vi "Sensor_Reads.vi"() -> ()   [LabVIEW 2020]
uses:
  <vilib>/Rock Robotics/WPI/ThirdParty/Phoenix-LabVIEW/Pigeon IMU/CTRE_PigeonIMU_TareType.ctl
  <vilib>/Rock Robotics/Network Tables/NT Read Number.vi
  Globals/Sensor_Values.vi
  Hardware/Drive/Drive_Hardware_Globals.vi
  Globals/Drive_Globals.vi
  <vilib>/Rock Robotics/Network Tables/NT Write Number.vi
  <vilib>/Rock Robotics/WPI/ThirdParty/Phoenix-LabVIEW/Pigeon IMU/CTRE_PigeonIMU_GetYPR.vi
  <vilib>/Rock Robotics/WPI/ThirdParty/Phoenix-LabVIEW/Motor Controller/Get/CTRE_Phoenix_MotorController_GetSelectedSensorData.vi
  Hardware/Climber/Climber_Hardware_Globals.vi
  <vilib>/Rock Robotics/WPI/ThirdParty/Phoenix-LabVIEW/CANCoder/Set/CTRE_Phoenix_CANcoder_SetPosition.vi
  Globals/Calibration_And_Constant_Globals.vi
  <vilib>/Rock Robotics/WPI/ThirdParty/Phoenix-LabVIEW/CANCoder/Get/CTRE_Phoenix_CANcoder_GetSensorData.vi
  Hardware/Cowl/Cowl_Hardware_Globals.vi
  Globals/Magazine_Globals.vi
  <vilib>/Rock Robotics/WPI/Utilities/WPI_GetSetVariantRefNum.vi
  Hardware/Flywheel/Flywheel_Hardware_Globals.vi
  Hardware/Turret/Turret_Hardware_Globals.vi
  <vilib>/Rock Robotics/WPI/ThirdParty/Phoenix-LabVIEW/Motor Controller/Get/CTRE_Phoenix_MotorController_GetPulseWidthAll.vi
  <vilib>/Rock Robotics/Network Tables/NT Read Boolean.vi
  Globals/Funnel_global.vi
  <vilib>/Rock Robotics/WPI/ThirdParty/Phoenix-LabVIEW/CANCoder/Set/CTRE_Phoenix_CANcoder_SetPositionToAbsolute.vi
  <vilib>/Rock Robotics/WPI/ThirdParty/Phoenix-LabVIEW/Motor Controller/Get/CTRE_Phoenix_MotorController_GetSupplyAndStatorCurrent_Enhanced.vi
panel:
  out "safe_to_move_turret?":bool
  in  "safe inner arm position for turret":i32
  in  "disable_limit_switch_zero_thing":bool
  out "Outer_Arm_Limit_Switch":bool=TRUE
  out "outer arm pulse width":i32
  out "inner arm pulse width":i32=578
  in  "inner arm pivot zero (ticks)":i32=-1151
  in  "outer arm pivot zero (ticks)":i32=921
  in  "reset_turret_position":bool
  out "turret position":i32
  in  "reset_cowl_position":bool
  in  "Cowl_Zero(deg)":dbl=61.6
  out "ball in funnel":bool
  in  "funnel current detect threshold":dbl=35.0
  in  "mag IR threshold":dbl=1.7
  out "limelight_distance_to_target":dbl=240.7612770897626
  out "Funnel_Supply_Current":dbl(graph)
  out "Mag IR Voltage":dbl=0.306396453
  in  "limelight mounting angle (deg)":dbl=36.64
  in  "height of the target (in)":dbl=104.0
  in  "height of robot (in)":dbl=37.625
  in  "Front_Right_Zero":dbl[](array[numeric])=[99.4, 331.43]
  out "front right raw":dbl=146.865234375
  out "FR mod":dbl=146.865234375
  in  "Front_Left_Zero":dbl[](array[numeric])=[338.818, 288.54]
  out "front left raw":dbl=111.357421875
  out "FL mod":dbl=111.357421875
  in  "Back_Left_Zero":dbl[](array[numeric])=[255.059, 271.84]
  out "back left raw":dbl=93.427734375
  out "BL mod":dbl=93.427734375
  in  "Back_Right_Zero":dbl[](array[numeric])=[182.197, 189.4]
  out "back right raw":dbl=195.29296875
  out "BR mod":dbl=195.29296875
  # "0th index is alpha, 1st index is beta"
  # "e"
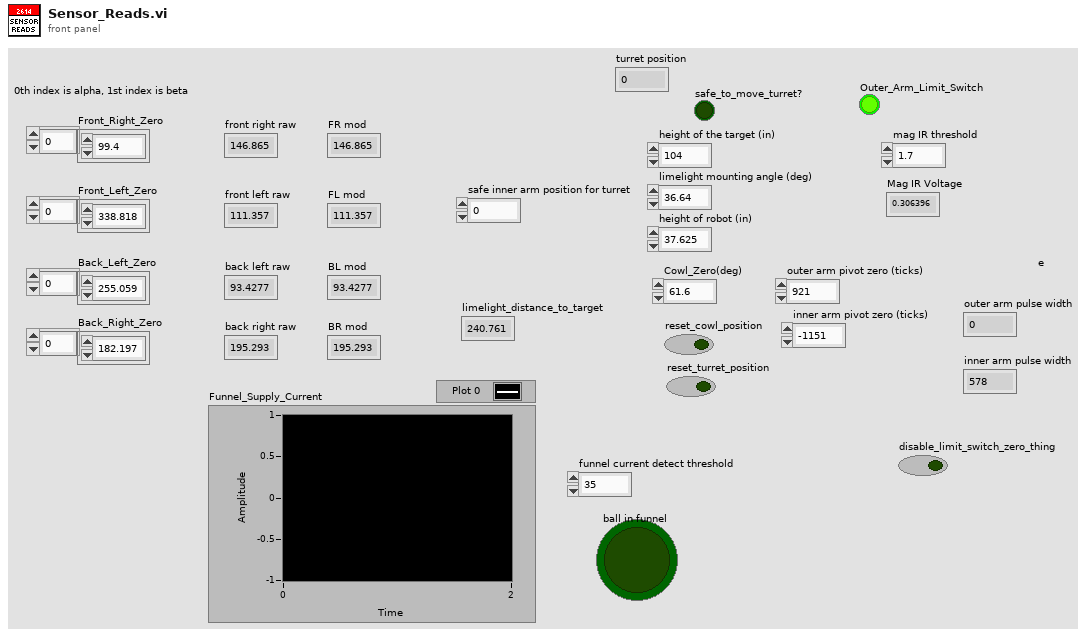
[diagram p1: front panel]
types:
  T1 = typedef "WPI_MotorControlDeviceRef.ctl" = cluster{"DeviceStatus":errorcluster, "Type":T2, "PWM":cluster{"PWM Channel":T3, "DeadBand":T4}, "CAN":cluster{"Device Number":u8, "SetOutput VI Ref":variant, "GetOutput VI Ref":variant, "Enable VI Ref":variant, "Disable VI Ref":variant, "Data":variant}, "Invert":bool, "DIO PWM":cluster{"PWM \"Enable\" Channel":T3, "DIOChannel":T5, "PWM Rate":dbl}}
  T2 = typedef "WPI_MotorControlType.ctl" = enum16{"PWM", "CAN", "DIO PWM"}
  T3 = typedef "FPGA_DIOPWMChannel.ctl" = enum8{"PWM 0", "PWM 1", "PWM 2", "PWM 3", "PWM 4", "PWM 5", "PWM 6", "PWM 7", "PWM 8", "PWM 9", "PWM MXP 0", "PWM MXP 1", "PWM MXP 2", "PWM MXP 3", "PWM MXP 4", "PWM MXP 5", "PWM MXP 6", "PWM MXP 7", "PWM MXP 8", "PWM MXP 9", "Invalid"}
  T4 = typedef "WPI_PWMDeadband.ctl" = cluster{"Name":string, "maxPositivePwm":i32, "minPositivePwm":i32, "centerPwm":i32, "maxNegativePwm":i32, "minNegativePwm":i32, "angularRange":u16}
  T5 = typedef "FPGA_DIOChannel.ctl" = enum8{"DIO 0", "DIO 1", "DIO 2", "DIO 3", "DIO 4", "DIO 5", "DIO 6", "DIO 7", "DIO 8", "DIO 9", "DIO MXP 0", "DIO MXP 1", "DIO MXP 2", "DIO MXP 3", "DIO MXP 4", "DIO MXP 5", "DIO MXP 6", "DIO MXP 7", "DIO MXP 8", "DIO MXP 9", "DIO MXP 10", "DIO MXP 11", "DIO MXP 12", "DIO MXP 13", "DIO MXP 14", "DIO MXP 15", "SPI Port CS1", "SPI Port CS2", "SPI Port CS3", "SPI Port MISO", "SPI Port MOSI", "Invalid"}
  T6 = typedef "CTRE_Phoenix_CANcoder_DeviceRef.ctl" = cluster{"DeviceStatus":errorcluster, "Device Number":u8, "Handle":u64, "UsageFrame":u32, "Library Path":path}
  T7 = typedef "CTRE_PigeonIMU_DeviceRef.ctl" = cluster{"DeviceStatus":errorcluster, "Device Number":u8, "Type":T8, "Device ID":u32, "Handle":u64, "UsageFrame":u32, "Library Path":path}
  T8 = typedef "CTRE_PigeonIMU_ConnectionType.ctl" = u32
  T9 = typedef "WPI_DigitalInputDevRef.ctl" = cluster{"DevStatus":errorcluster, "DIO Channel":T5}
  T10 = typedef "WPI_AnalogChannelDevRef.ctl" = cluster{"DevStatus":errorcluster, "Analog Channel":T11}
  T11 = typedef "FPGA_AIChannel.ctl" = enum8{"AI 0", "AI 1", "AI 2", "AI 3", "AI MXP 0", "AI MXP 1", "AI MXP 2", "AI MXP 3", "Invalid"}
  T12 = typedef "CTRE_PigeonIMU_TareType.ctl" = u8
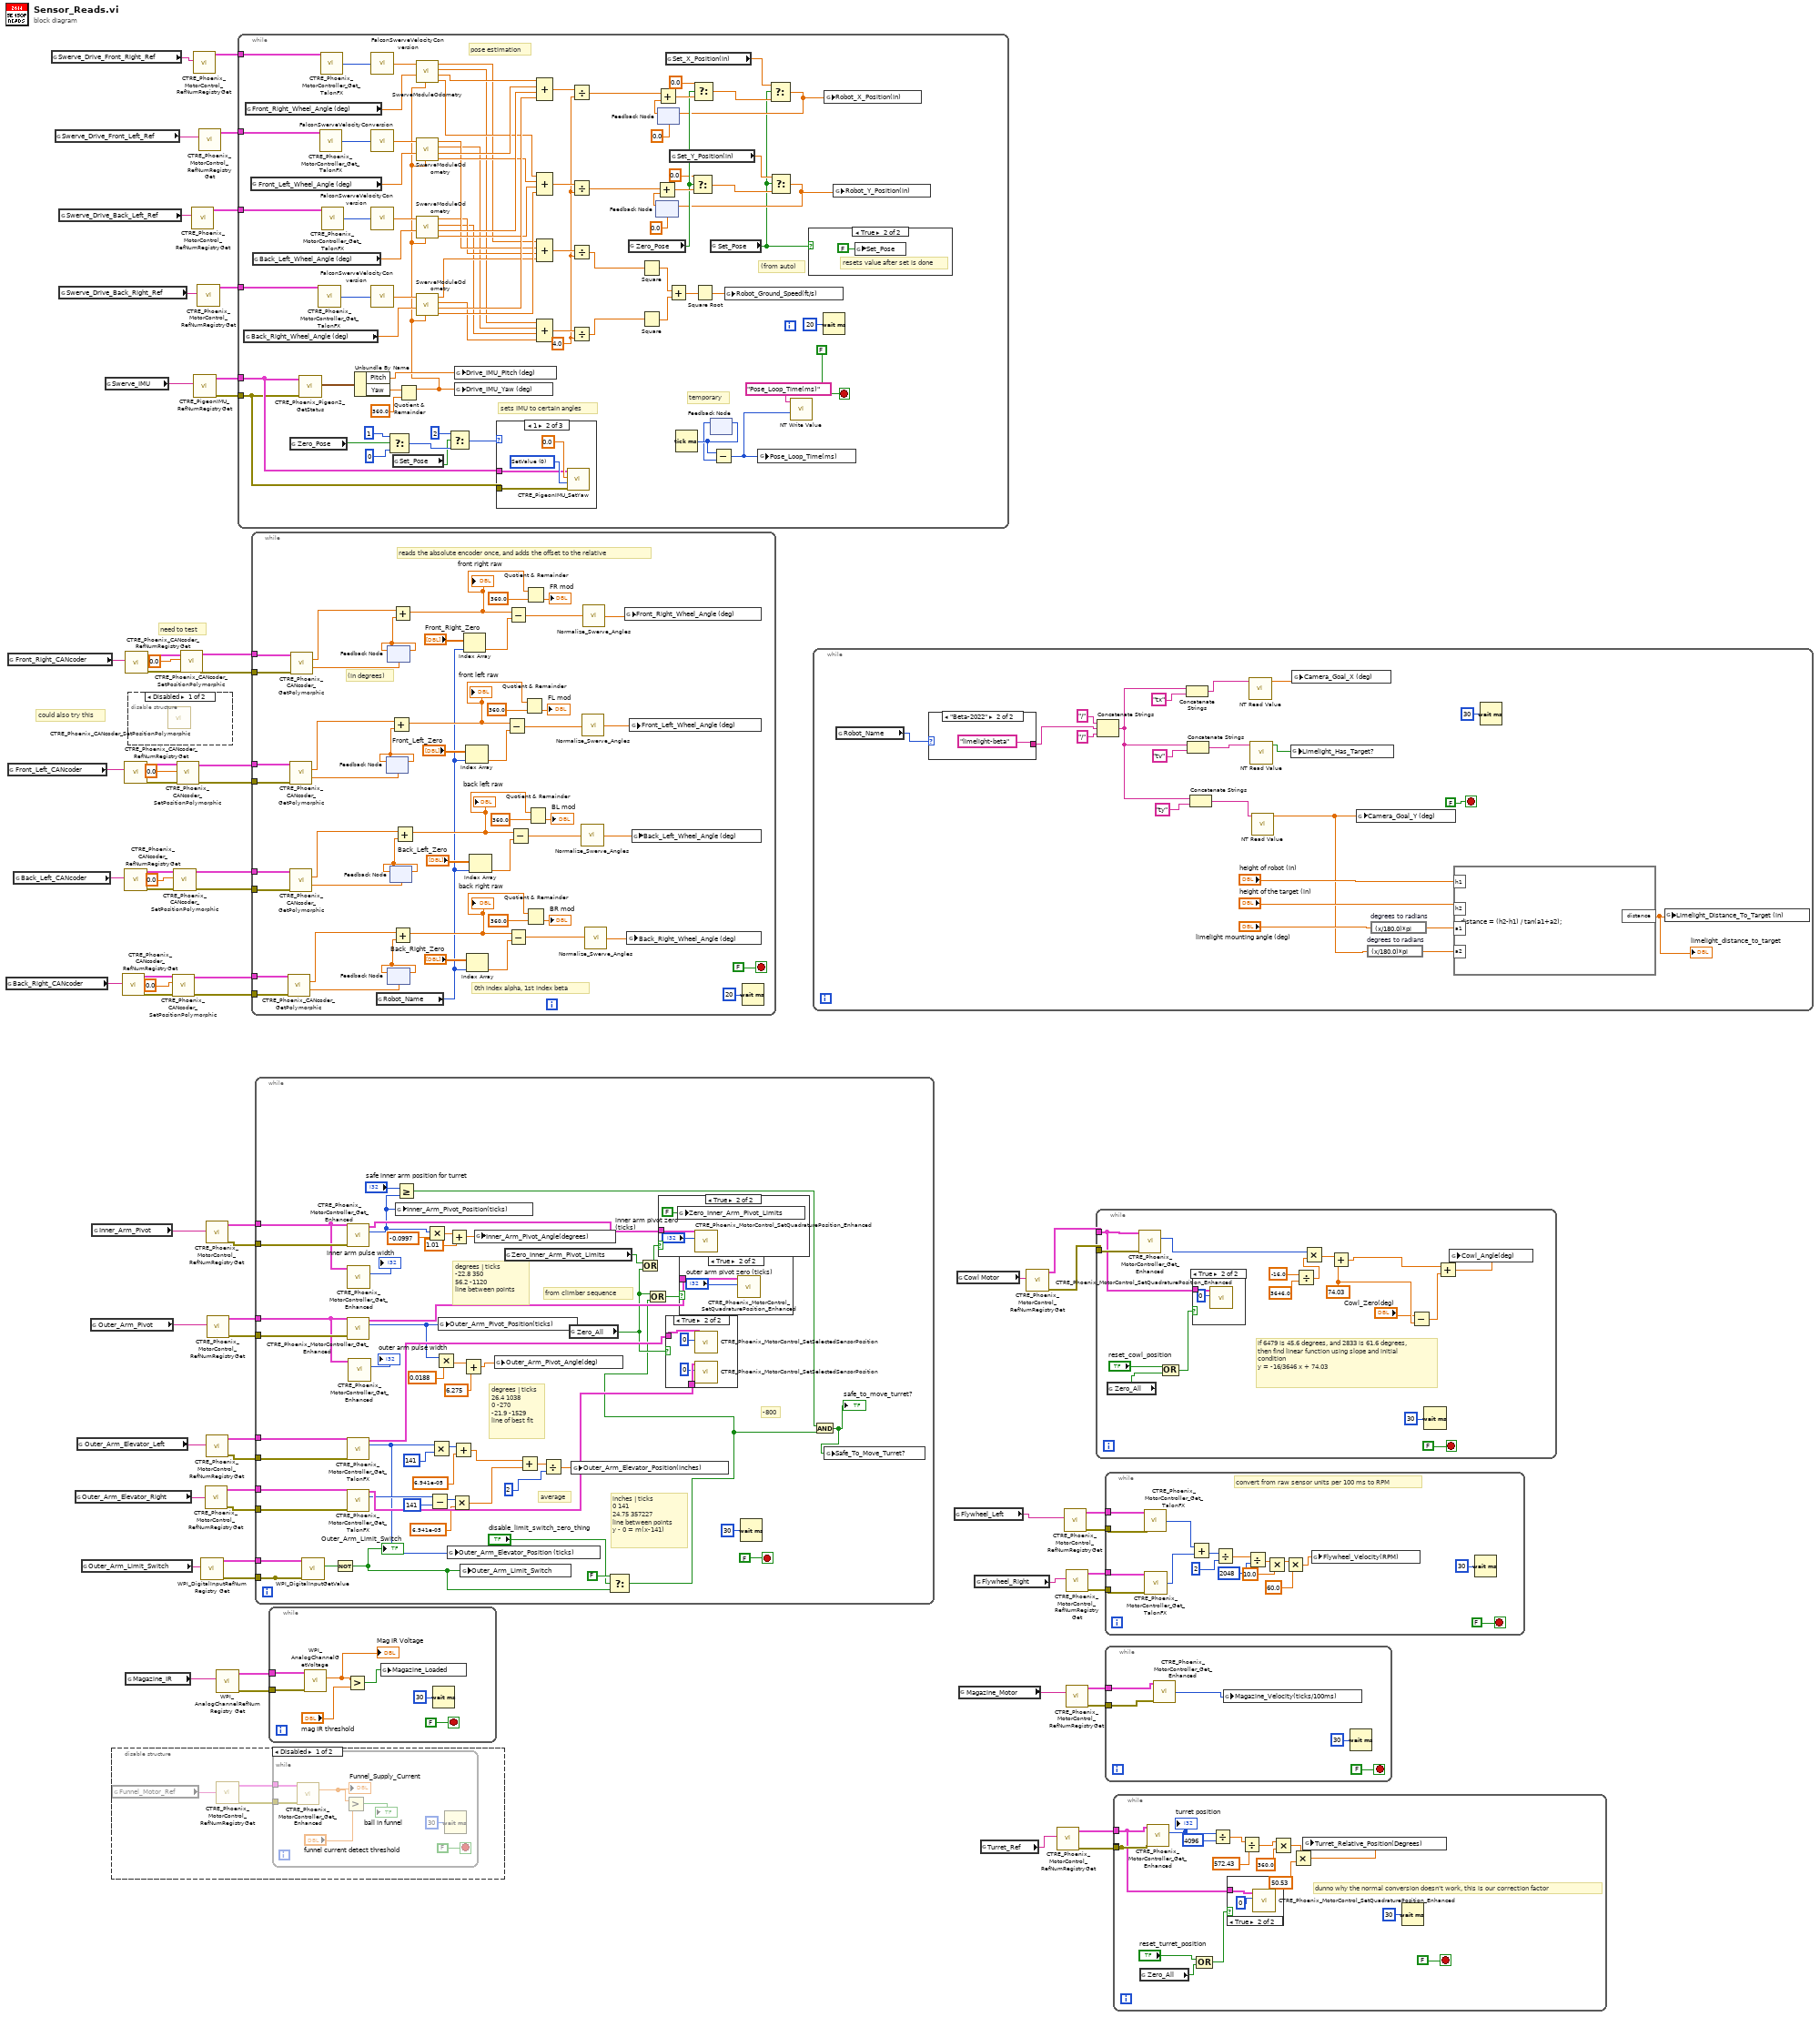
[diagram p0: block diagram]
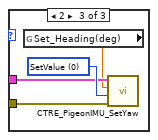
[diagram p10: hidden frame]
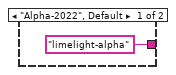
[diagram p12: hidden frame]
diagram:
  # "could also try this"
  # "need to test"
  n1 = global read "Drive_Hardware_Globals.vi" "Back_Right_CANcoder"() -> (w54:string)
  n2 = global read "Drive_Hardware_Globals.vi" "Front_Right_CANcoder"() -> (w57:string)
  n3 = global read "Drive_Hardware_Globals.vi" "Front_Left_CANcoder"() -> (w56:string)
  n4 = global read "Drive_Hardware_Globals.vi" "Back_Left_CANcoder"() -> (w55:string)
  n5 = global read "Drive_Hardware_Globals.vi" "Swerve_Drive_Front_Right_Ref"() -> (w58:string)
  n6 = global read "Drive_Hardware_Globals.vi" "Swerve_Drive_Front_Left_Ref"() -> (w59:string)
  n7 = global read "Drive_Hardware_Globals.vi" "Swerve_Drive_Back_Left_Ref"() -> (w68:string)
  n8 = global read "Drive_Hardware_Globals.vi" "Swerve_Drive_Back_Right_Ref"() -> (w67:string)
  n9 = global read "Climber_Hardware_Globals.vi" "Outer_Arm_Elevator_Right"() -> (w32:string)
  n10 = global read "Climber_Hardware_Globals.vi" "Outer_Arm_Elevator_Left"() -> (w33:string)
  n11 = global read "Climber_Hardware_Globals.vi" "Outer_Arm_Limit_Switch"() -> (w3:string)
  n12 = global read "Climber_Hardware_Globals.vi" "Outer_Arm_Pivot"() -> (w22:string)
  n13 = global read "Climber_Hardware_Globals.vi" "Inner_Arm_Pivot"() -> (w31:string)
  n14 = global read "Drive_Hardware_Globals.vi" "Swerve_IMU"() -> (w62:string)
  n15 = disable-structure shown="Disabled" {
    frame Disabled {
      n16 = global read "Funnel_global.vi" "Funnel_Motor_Ref"() -> (w71:string)
      n17 = call <vilib>:"CTRE_Phoenix_MotorControl_RefNumRegistryGet.vi"("refnum name"=w71) -> ("error out"=w69:errorcluster, "PhoenixMotorControlDevRef"=w70:T1)  [unwired: 9 in]
      n18 = while {
        tunnel: w70 -> [w76]
        tunnel: w69 -> [w75]
        stop <- FALSE stop-if-true
        n19 = call-poly <vilib>:"CTRE_Phoenix_MotorController_Get_Enhanced.vi"("PhoenixMotorControlDevRef"=w76, "error in"=w75) -> ("Supply Current"=w74:dbl)  [unwired: 10 in, 3 out]
        "Funnel_Supply_Current" <- w74
        n20 = Greater?(x=w74, y="funnel current detect threshold") -> (0:→"ball in funnel":bool)
        n21 = Wait (ms)(milliseconds to wait=u32 30) -> ()  [unwired: 1 out]
      }
    }
    frame Enabled {
    }
  }
  n22 = call <vilib>:"CTRE_Phoenix_CANcoder_RefNumRegistryGet.vi"("refnum name"=w54) -> ("error out"=w40:errorcluster, "CTRE_CANcoder_DeviceRef"=w43:T6)  [unwired: 9 in]
  n23 = call <vilib>:"CTRE_Phoenix_CANcoder_RefNumRegistryGet.vi"("refnum name"=w56) -> ("error out"=w48:errorcluster, "CTRE_CANcoder_DeviceRef"=w51:T6)  [unwired: 9 in]
  n24 = call <vilib>:"CTRE_Phoenix_CANcoder_RefNumRegistryGet.vi"("refnum name"=w55) -> ("error out"=w45:errorcluster, "CTRE_CANcoder_DeviceRef"=w47:T6)  [unwired: 9 in]
  n25 = call <vilib>:"CTRE_Phoenix_CANcoder_RefNumRegistryGet.vi"("refnum name"=w57) -> ("error out"=w53:errorcluster, "CTRE_CANcoder_DeviceRef"=w52:T6)  [unwired: 9 in]
  n26 = global read "Magazine_Globals.vi" "Magazine_IR"() -> (w20:string)
  n27 = disable-structure shown="Disabled" {
    frame Disabled {
      n28 = call-poly <vilib>:"CTRE_Phoenix_CANcoder_SetPositionPolymorphic.vi"() -> ()  [unwired: 10 in, 2 out]
    }
    frame Enabled {
    }
  }
  n29 = call-poly <vilib>:"CTRE_Phoenix_CANcoder_SetPositionPolymorphic.vi"("error in (no error)"=w40, "Position"=0.0, "CTRE_CANcoder_DeviceRef"=w43) -> ("error out"=w41:errorcluster, "CTRE_CANcoder_DeviceRef"=w42:T6)  [unwired: 7 in]
  n30 = call-poly <vilib>:"CTRE_Phoenix_CANcoder_SetPositionPolymorphic.vi"("error in (no error)"=w45, "Position"=0.0, "CTRE_CANcoder_DeviceRef"=w47) -> ("error out"=w44:errorcluster, "CTRE_CANcoder_DeviceRef"=w46:T6)  [unwired: 7 in]
  n31 = call-poly <vilib>:"CTRE_Phoenix_CANcoder_SetPositionPolymorphic.vi"("error in (no error)"=w48, "Position"=0.0, "CTRE_CANcoder_DeviceRef"=w51) -> ("error out"=w49:errorcluster, "CTRE_CANcoder_DeviceRef"=w50:T6)  [unwired: 7 in]
  n32 = call-poly <vilib>:"CTRE_Phoenix_CANcoder_SetPositionPolymorphic.vi"("error in (no error)"=w53, "Position"=0.0, "CTRE_CANcoder_DeviceRef"=w52) -> ("error out"=w38:errorcluster, "CTRE_CANcoder_DeviceRef"=w39:T6)  [unwired: 7 in]
  n33 = call <vilib>:"CTRE_Phoenix_MotorControl_RefNumRegistryGet.vi"("refnum name"=w68) -> ("PhoenixMotorControlDevRef"=w64:T1)  [unwired: 9 in, 1 out]
  n34 = call <vilib>:"CTRE_Phoenix_MotorControl_RefNumRegistryGet.vi"("refnum name"=w58) -> ("PhoenixMotorControlDevRef"=w66:T1)  [unwired: 9 in, 1 out]
  n35 = call <vilib>:"CTRE_PigeonIMU_RefNumRegistryGet.vi"("refnum name"=w62) -> ("error out"=w60:errorcluster, "PigeonIMUDevRef"=w61:T7)  [unwired: 9 in]
  n36 = call <vilib>:"CTRE_Phoenix_MotorControl_RefNumRegistryGet.vi"("refnum name"=w67) -> ("PhoenixMotorControlDevRef"=w63:T1)  [unwired: 9 in, 1 out]
  n37 = call <vilib>:"CTRE_Phoenix_MotorControl_RefNumRegistryGet.vi"("refnum name"=w59) -> ("PhoenixMotorControlDevRef"=w65:T1)  [unwired: 9 in, 1 out]
  n38 = call <vilib>:"WPI_DigitalInputRefNum Registry Get.vi"("refnum name"=w3) -> ("error out"=w1:errorcluster, "DigitalInputDevRef"=w2:T9)  [unwired: 9 in]
  n39 = call <vilib>:"CTRE_Phoenix_MotorControl_RefNumRegistryGet.vi"("refnum name"=w32) -> ("error out"=w26:errorcluster, "PhoenixMotorControlDevRef"=w25:T1)  [unwired: 9 in]
  n40 = call <vilib>:"CTRE_Phoenix_MotorControl_RefNumRegistryGet.vi"("refnum name"=w31) -> ("error out"=w24:errorcluster, "PhoenixMotorControlDevRef"=w23:T1)  [unwired: 9 in]
  n41 = call <vilib>:"CTRE_Phoenix_MotorControl_RefNumRegistryGet.vi"("refnum name"=w33) -> ("error out"=w28:errorcluster, "PhoenixMotorControlDevRef"=w27:T1)  [unwired: 9 in]
  n42 = call <vilib>:"CTRE_Phoenix_MotorControl_RefNumRegistryGet.vi"("refnum name"=w22) -> ("error out"=w30:errorcluster, "PhoenixMotorControlDevRef"=w29:T1)  [unwired: 9 in]
  n43 = call <vilib>:"WPI_AnalogChannelRefNum Registry Get.vi"("refnum name"=w20) -> ("error out"=w18:errorcluster, "AIDeviceRef"=w19:T10)  [unwired: 9 in]
  n44 = while {
    tunnel: w66 -> [w159]
    tunnel: w65 -> [w158]
    tunnel: w64 -> [w157]
    tunnel: w63 -> [w156]
    tunnel: w61 -> [w106]
    tunnel: w60 -> [w105]
    stop <- FALSE stop-if-true
    w91 = 4.0 ("y")
    # "sets IMU to certain angles"
    # "(from auto)"
    # "temporary"
    # "pose estimation"
    n45 = global read "Sensor_Values.vi" "Back_Right_Wheel_Angle (deg)"() -> (w147:dbl)
    n46 = global read "Sensor_Values.vi" "Front_Right_Wheel_Angle (deg)"() -> (w108:dbl)
    n47 = global read "Sensor_Values.vi" "Front_Left_Wheel_Angle (deg)"() -> (w107:dbl)
    n48 = global read "Sensor_Values.vi" "Back_Left_Wheel_Angle (deg)"() -> (w146:dbl)
    n49 = global read "Drive_Globals.vi" "Zero_Pose"() -> (w86:bool)
    n50 = call-poly <vilib>:"CTRE_Phoenix_Pigeon2_GetStatus.vi"("error in (no error)"=w105, "PigeonIMUDevRef"=w106) -> ("Yaw Pitch Roll"=w90:cluster{"Yaw":dbl, "Pitch":dbl, "Roll":dbl})  [unwired: 7 in, 2 out]
    n51 = call-poly <vilib>:"CTRE_Phoenix_MotorController_Get_TalonFX.vi"("PhoenixMotorControlDevRef"=w156) -> ("Velocity (Raw Sensor Units per 100 ms)"=w152:i32)  [unwired: 11 in, 3 out]
    n52 = call-poly <vilib>:"CTRE_Phoenix_MotorController_Get_TalonFX.vi"("PhoenixMotorControlDevRef"=w158) -> ("Velocity (Raw Sensor Units per 100 ms)"=w154:i32)  [unwired: 11 in, 3 out]
    n53 = call-poly <vilib>:"CTRE_Phoenix_MotorController_Get_TalonFX.vi"("PhoenixMotorControlDevRef"=w159) -> ("Velocity (Raw Sensor Units per 100 ms)"=w155:i32)  [unwired: 11 in, 3 out]
    n54 = call-poly <vilib>:"CTRE_Phoenix_MotorController_Get_TalonFX.vi"("PhoenixMotorControlDevRef"=w157) -> ("Velocity (Raw Sensor Units per 100 ms)"=w153:i32)  [unwired: 11 in, 3 out]
    n55 = Unbundle By Name(w90) -> ("Pitch"=w80:dbl, "Yaw"=w89:dbl)
    n56 = call "FalconSwerveVelocityConversion.vi"("Velocity (Raw Sensor Units per 100 ms)"=w155) -> ("Velocity (ft/s)"=w151:dbl)
    n57 = call "FalconSwerveVelocityConversion.vi"("Velocity (Raw Sensor Units per 100 ms)"=w154) -> ("Velocity (ft/s)"=w150:dbl)
    n58 = call "FalconSwerveVelocityConversion.vi"("Velocity (Raw Sensor Units per 100 ms)"=w153) -> ("Velocity (ft/s)"=w149:dbl)
    n59 = call "FalconSwerveVelocityConversion.vi"("Velocity (Raw Sensor Units per 100 ms)"=w152) -> ("Velocity (ft/s)"=w148:dbl)
    n60 = Select(t=1, s=w86, f=0 ("Velocity (Raw Sensor Units per 100 ms)")) -> (s? t:f=w84:i32)
    n61 = global read "Drive_Globals.vi" "Set_Pose"() -> (w82:bool)
    n62 = Quotient & Remainder(x=w89, y=360.0) -> (x-y*floor(x/y)=w79:dbl)  [unwired: 1 out]
    n63 = call "SwerveModuleOdometry.vi"("Robot Heading(deg)"=w79, "Wheel Azimuth (deg)"=w108, "Velocity (ft/s)"=w151) -> ("Delta Y (in)"=w141:dbl, "Delta X (in)"=w145:dbl, "Velocity Y (ft/s)"=w127:dbl, "Velocity X (ft/s)"=w131:dbl)  [unwired: 3 in]
    n64 = call "SwerveModuleOdometry.vi"("Robot Heading(deg)"=w79, "Wheel Azimuth (deg)"=w107, "Velocity (ft/s)"=w150) -> ("Delta Y (in)"=w140:dbl, "Delta X (in)"=w144:dbl, "Velocity Y (ft/s)"=w126:dbl, "Velocity X (ft/s)"=w130:dbl)  [unwired: 3 in]
    n65 = call "SwerveModuleOdometry.vi"("Robot Heading(deg)"=w79, "Wheel Azimuth (deg)"=w146, "Velocity (ft/s)"=w149) -> ("Delta Y (in)"=w139:dbl, "Delta X (in)"=w143:dbl, "Velocity Y (ft/s)"=w125:dbl, "Velocity X (ft/s)"=w129:dbl)  [unwired: 3 in]
    n66 = call "SwerveModuleOdometry.vi"("Robot Heading(deg)"=w79, "Wheel Azimuth (deg)"=w147, "Velocity (ft/s)"=w148) -> ("Delta Y (in)"=w138:dbl, "Delta X (in)"=w142:dbl, "Velocity Y (ft/s)"=w124:dbl, "Velocity X (ft/s)"=w128:dbl)  [unwired: 3 in]
    n67 = Select(t=2, s=w82, f=w84) -> (s? t:f=w81:i32)
    n68 = global write "Sensor_Values.vi" "Drive_IMU_Pitch (deg)"(w80) -> ()
    n69 = global write "Sensor_Values.vi" "Drive_IMU_Yaw (deg)"(w79) -> ()
    n70 = case shown="1" w81 {
      tunnel: w106 -> [_ w161 w166]
      tunnel: w105 -> [_ w160 w165]
      frame 0, Default {
      }
      frame 1 {
        w162 = T12 0 items=["SetValue"=0, "AddOffset"=1, "MatchCompass"=2, "SetOffset"=255] ("TareType (SetValue)")
        n71 = call <vilib>:"CTRE_PigeonIMU_SetYaw.vi"("error in (no error)"=w160, "TareType (SetValue)"=w162, "Value"=0.0, "PigeonIMUDevRef"=w161) -> ()  [unwired: 6 in, 2 out]
      }
      frame 2 {
        w167 = T12 0 items=["SetValue"=0, "AddOffset"=1, "MatchCompass"=2, "SetOffset"=255] ("TareType (SetValue)")
        n72 = global read "Drive_Globals.vi" "Set_Heading(deg)"() -> (w164:dbl)
        n73 = call <vilib>:"CTRE_PigeonIMU_SetYaw.vi"("error in (no error)"=w165, "TareType (SetValue)"=w167, "Value"=w164, "PigeonIMUDevRef"=w166) -> ()  [unwired: 6 in, 2 out]
      }
    }
    n74 = Compound Arithmetic op=ADD(w145, w144, w143, w142) -> (w123:dbl)
    n75 = Compound Arithmetic op=ADD(w141, w140, w139, w138) -> (w122:dbl)
    n76 = Compound Arithmetic op=ADD(w131, w130, w129, w128) -> (w121:dbl)
    n77 = Compound Arithmetic op=ADD(w127, w126, w125, w124) -> (w120:dbl)
    n78 = Divide(x=w123, y=w91) -> (x/y=w101:dbl)
    n79 = Divide(x=w122, y=w91) -> (x/y=w119:dbl)
    n80 = Divide(x=w121, y=w91) -> (x/y=w110:dbl)
    n81 = Divide(x=w120, y=w91) -> (x/y=w109:dbl)
    n82 = global read "Drive_Globals.vi" "Zero_Pose"() -> (w102:bool)
    n83 = Square(x=w110) -> (x^2=w118:dbl)
    n84 = Square(x=w109) -> (x^2=w117:dbl)
    n85 = feedback #1(0.0) -> (w134:dbl)
    n86 = Add(x=w119, y=w134) -> (x+y=w104:dbl)
    n87 = feedback #2(0.0) -> (w135:dbl)
    n88 = Add(x=w101, y=w135) -> (x+y=w103:dbl)
    n89 = global read "Drive_Globals.vi" "Set_X_Position(in)"() -> (w94:dbl)
    n90 = Add(x=w118, y=w117) -> (x+y=w116:dbl)
    n91 = global read "Drive_Globals.vi" "Set_Y_Position(in)"() -> (w93:dbl)
    n92 = Tick Count (ms)() -> (millisecond timer value=w114:u32)
    n93 = Select(t=0.0, s=w102, f=w104) -> (s? t:f=w98:dbl)
    n94 = Select(t=0.0, s=w102, f=w103) -> (s? t:f=w97:dbl)
    n95 = Square Root(x=w116) -> (sqrt(x)=w115:dbl)
    n96 = global read "Drive_Globals.vi" "Set_Pose"() -> (w92:bool)
    n97 = feedback-in #3(w114) -> ()
    n98 = feedback #3() -> (w113:u32)  [unwired: 1 in]
    n99 = Subtract(x=w114, y=w113) -> (x-y=w112:u32)
    n100 = global write "Sensor_Values.vi" "Robot_Ground_Speed(ft/s)"(w115) -> ()
    n101 = global write "Sensor_Values.vi" "Pose_Loop_Time(ms)"(w112) -> ()
    n102 = Select(t=w94, s=w92, f=w97) -> (s? t:f=w96:dbl)
    n103 = feedback-in #2(w96) -> ()
    n104 = Select(t=w93, s=w92, f=w98) -> (s? t:f=w95:dbl)
    n105 = feedback-in #1(w95) -> ()
    n106 = call-poly <vilib>:"NT Write Value.vi"("Numeric"=w112, "Name"="Pose_Loop_Time(ms)") -> ()  [unwired: 9 in, 1 out]
    n107 = case shown="True" w92 {
      frame False {
      }
      frame True {
        # "resets value after set is done"
        n108 = global write "Drive_Globals.vi" "Set_Pose"(FALSE ("Set_Pose")) -> ()
      }
    }
    n109 = Wait (ms)(milliseconds to wait=u32 20) -> ()  [unwired: 1 out]
    n110 = global write "Sensor_Values.vi" "Robot_X_Position(in)"(w96) -> ()
    n111 = global write "Sensor_Values.vi" "Robot_Y_Position(in)"(w95) -> ()
  }
  n112 = while {
    tunnel: w42 -> [w201]
    tunnel: w41 -> [w200]
    tunnel: w46 -> [w199]
    tunnel: w44 -> [w198]
    tunnel: w50 -> [w197]
    tunnel: w49 -> [w196]
    tunnel: w39 -> [w195]
    tunnel: w38 -> [w194]
    stop <- FALSE stop-if-true
    # "0th index alpha, 1st index beta"
    # "reads the absolute encoder once, and adds the offset to the relative"
    # "(in degrees)"
    n113 = call-poly <vilib>:"CTRE_Phoenix_CANcoder_GetPolymorphic.vi"("CTRE_CANcoder_DeviceRef"=w201, "error in"=w200) -> ("Position"=w193:dbl, "Absolute Position"=w192:dbl)  [unwired: 9 in, 3 out]
    n114 = call-poly <vilib>:"CTRE_Phoenix_CANcoder_GetPolymorphic.vi"("CTRE_CANcoder_DeviceRef"=w197, "error in"=w196) -> ("Position"=w189:dbl, "Absolute Position"=w188:dbl)  [unwired: 9 in, 3 out]
    n115 = call-poly <vilib>:"CTRE_Phoenix_CANcoder_GetPolymorphic.vi"("CTRE_CANcoder_DeviceRef"=w199, "error in"=w198) -> ("Position"=w191:dbl, "Absolute Position"=w190:dbl)  [unwired: 9 in, 3 out]
    n116 = call-poly <vilib>:"CTRE_Phoenix_CANcoder_GetPolymorphic.vi"("CTRE_CANcoder_DeviceRef"=w195, "error in"=w194) -> ("Position"=w187:dbl, "Absolute Position"=w186:dbl)  [unwired: 9 in, 3 out]
    n117 = global read "Calibration_And_Constant_Globals.vi" "Robot_Name"() -> (w173:enum16{"Alpha-2022", "Beta-2022"})
    n118 = feedback #4(w188) -> (w210:dbl)
    n119 = feedback-in #4(w210) -> ()
    n120 = feedback #5(w186) -> (w217:dbl)
    n121 = feedback-in #5(w217) -> ()
    n122 = feedback #6(w192) -> (w202:dbl)
    n123 = feedback-in #6(w202) -> ()
    n124 = feedback #7(w190) -> (w209:dbl)
    n125 = feedback-in #7(w209) -> ()
    n126 = Add(x=w189, y=w210) -> (x+y=w211:dbl)
    "front left raw" <- w211
    n127 = Add(x=w187, y=w217) -> (x+y=w216:dbl)
    "front right raw" <- w216
    n128 = Add(x=w193, y=w202) -> (x+y=w203:dbl)
    "back right raw" <- w203
    n129 = Add(x=w191, y=w209) -> (x+y=w208:dbl)
    "back left raw" <- w208
    n130 = Index Array(array="Front_Right_Zero", index=w173) -> (element=w172:dbl)
    n131 = Index Array(array="Front_Left_Zero", index=w173) -> (element=w171:dbl)
    n132 = Index Array(array="Back_Right_Zero", index=w173) -> (element=w169:dbl)
    n133 = Index Array(array="Back_Left_Zero", index=w173) -> (element=w170:dbl)
    n134 = Subtract(x=w211, y=w171) -> (x-y=w183:dbl)
    n135 = Subtract(x=w216, y=w172) -> (x-y=w185:dbl)
    n136 = Subtract(x=w203, y=w169) -> (x-y=w181:dbl)
    n137 = Subtract(x=w208, y=w170) -> (x-y=w182:dbl)
    n138 = Quotient & Remainder(x=w211, y=360.0 ("x+y")) -> (x-y*floor(x/y)=→"FL mod":dbl)  [unwired: 1 out]
    n139 = Quotient & Remainder(x=w216, y=360.0 ("x+y")) -> (x-y*floor(x/y)=→"FR mod":dbl)  [unwired: 1 out]
    n140 = Quotient & Remainder(x=w203, y=360.0 ("x+y")) -> (x-y*floor(x/y)=→"BR mod":dbl)  [unwired: 1 out]
    n141 = Quotient & Remainder(x=w208, y=360.0 ("x+y")) -> (x-y*floor(x/y)=→"BL mod":dbl)  [unwired: 1 out]
    n142 = call "Normalize_Swerve_Angles.vi"("input angle [0, 360]"=w182) -> ("output angle [-180, 180]"=w179:dbl)
    n143 = call "Normalize_Swerve_Angles.vi"("input angle [0, 360]"=w183) -> ("output angle [-180, 180]"=w180:dbl)
    n144 = call "Normalize_Swerve_Angles.vi"("input angle [0, 360]"=w185) -> ("output angle [-180, 180]"=w184:dbl)
    n145 = call "Normalize_Swerve_Angles.vi"("input angle [0, 360]"=w181) -> ("output angle [-180, 180]"=w178:dbl)
    n146 = global write "Sensor_Values.vi" "Front_Right_Wheel_Angle (deg)"(w184) -> ()
    n147 = global write "Sensor_Values.vi" "Back_Right_Wheel_Angle (deg)"(w178) -> ()
    n148 = global write "Sensor_Values.vi" "Front_Left_Wheel_Angle (deg)"(w180) -> ()
    n149 = global write "Sensor_Values.vi" "Back_Left_Wheel_Angle (deg)"(w179) -> ()
    n150 = Wait (ms)(milliseconds to wait=u32 20) -> ()  [unwired: 1 out]
  }
  n151 = while {
    tunnel: w30 -> [w268]
    tunnel: w29 -> [w257]
    tunnel: w28 -> [w267]
    tunnel: w27 -> [w266]
    tunnel: w26 -> [w265]
    tunnel: w25 -> [w264]
    tunnel: w24 -> [w263]
    tunnel: w23 -> [w258]
    tunnel: w2 -> [w232]
    tunnel: [w231] -> _
    tunnel: w1 -> [w231]
    stop <- FALSE stop-if-true
    # "-800"
    # "from climber sequence"
    # "degrees | ticks\n-22.8 350\n56.2 -1120\nline between points"
    # "inches | ticks\n0 141\n24.75 357227\nline between points\ny - 0 = m(x-141)"
    # "degrees | ticks\n26.4 1038\n0 -270\n-21.9 -1529\nline of best fit"
    # "average"
    n152 = call <vilib>:"WPI_DigitalInputGetValue.vi"("error in (no error)"=w231, "DigitalInputDevRef"=w232) -> ("Value"=w230:bool)  [unwired: 7 in, 2 out]
    n153 = Not(x=w230) -> (.not. x?=w227:bool)
    "Outer_Arm_Limit_Switch" <- w227
    n154 = call-poly <vilib>:"CTRE_Phoenix_MotorController_Get_Enhanced.vi"("PhoenixMotorControlDevRef"=w258, "error in"=w263) -> ("PhoenixMotorControlDevRef"=w262:T1, "Position (Raw Sensor Units)"=w224:i32)  [unwired: 10 in, 2 out]
    n155 = call-poly <vilib>:"CTRE_Phoenix_MotorController_Get_Enhanced.vi"("PhoenixMotorControlDevRef"=w257, "error in"=w268) -> ("PhoenixMotorControlDevRef"=w261:T1, "Position (Raw Sensor Units)"=w250:i32)  [unwired: 10 in, 2 out]
    n156 = call-poly <vilib>:"CTRE_Phoenix_MotorController_Get_TalonFX.vi"("PhoenixMotorControlDevRef"=w266, "error in"=w267) -> ("PhoenixMotorControlDevRef"=w260:T1, "Position (Raw Sensor Units)"=w236:i32)  [unwired: 10 in, 2 out]
    n157 = call-poly <vilib>:"CTRE_Phoenix_MotorController_Get_TalonFX.vi"("PhoenixMotorControlDevRef"=w264, "error in"=w265) -> ("PhoenixMotorControlDevRef"=w259:T1, "Position (Raw Sensor Units)"=w243:i32)  [unwired: 10 in, 2 out]
    n158 = call-poly <vilib>:"CTRE_Phoenix_MotorController_Get_Enhanced.vi"("PhoenixMotorControlDevRef"=w258) -> ("Pulse Width Position"=→"inner arm pulse width":i32)  [unwired: 9 in, 5 out]
    n159 = call-poly <vilib>:"CTRE_Phoenix_MotorController_Get_Enhanced.vi"("PhoenixMotorControlDevRef"=w257) -> ("Pulse Width Position"=→"outer arm pulse width":i32)  [unwired: 9 in, 5 out]
    n160 = Greater Or Equal?(x="safe inner arm position for turret", y=w224) -> (x >= y?=w221:bool)
    n161 = global write "Sensor_Values.vi" "Inner_Arm_Pivot_Position(ticks)"(w224) -> ()
    n162 = Multiply(x=w224, y=-0.0997) -> (x*y=w253:dbl)
    n163 = Subtract(x=w243, y=141) -> (x-y=w244:i32)
    n164 = Multiply(x=w236, y=141) -> (x*y=w245:i32)
    n165 = Multiply(x=w250, y=0.0188) -> (x*y=w248:dbl)
    n166 = global write "Sensor_Values.vi" "Outer_Arm_Pivot_Position(ticks)"(w250) -> ()
    n167 = global write "Sensor_Values.vi" "Outer_Arm_Elevator_Position (ticks)"(w236) -> ()
    n168 = Add(x=w253, y=1.01) -> (x+y=w251:dbl)
    n169 = Multiply(x=w244, y=6.941e-05 ("x")) -> (x*y=w241:dbl)
    n170 = Add(x=w245, y=6.941e-05 ("x")) -> (x+y=w242:dbl)
    n171 = global write "Sensor_Values.vi" "Outer_Arm_Limit_Switch"(w227) -> ()
    n172 = Add(x=w248, y=6.275) -> (x+y=w246:dbl)
    n173 = global write "Sensor_Values.vi" "Inner_Arm_Pivot_Angle(degrees)"(w251) -> ()
    n174 = global write "Sensor_Values.vi" "Outer_Arm_Pivot_Angle(deg)"(w246) -> ()
    n175 = global read "Calibration_And_Constant_Globals.vi" "Zero_Inner_Arm_Pivot_Limits"() -> (w234:bool)
    n176 = Add(x=w242, y=w241) -> (x+y=w271:dbl)
    n177 = Divide(x=w271, y=2) -> (x/y=w235:dbl)
    n178 = global read "Calibration_And_Constant_Globals.vi" "Zero_All"() -> (w229:bool)
    n179 = global write "Sensor_Values.vi" "Outer_Arm_Elevator_Position(inches)"(w235) -> ()
    n180 = Select(t=FALSE, s="disable_limit_switch_zero_thing", f=w227) -> (s? t:f=w222:bool)
    n181 = Or(x=w234, y=w229) -> (x .or. y?=w233:bool)
    n182 = Or(x=w229, y=w222) -> (x .or. y?=w228:bool)
    n183 = case shown="True" w233 {
      tunnel: w262 -> [_ w281]
      frame False {
      }
      frame True {
        n184 = global write "Calibration_And_Constant_Globals.vi" "Zero_Inner_Arm_Pivot_Limits"(FALSE ("Zero_Inner_Arm_Pivot_Limits")) -> ()
        n185 = call <vilib>:"CTRE_Phoenix_MotorControl_SetQuadraturePosition_Enhanced.vi"("New Position"="inner arm pivot zero (ticks)", "PhoenixMotorControlDevRef"=w281) -> ()  [unwired: 8 in, 2 out]
      }
    }
    n186 = case shown="True" w229 {
      tunnel: w260 -> [_ w278]
      tunnel: w259 -> [_ w277]
      frame False {
      }
      frame True {
        n187 = call <vilib>:"CTRE_Phoenix_MotorControl_SetSelectedSensorPosition.vi"("New Sensor Position"=0 ("New Position"), "PhoenixMotorControlDevRef"=w278) -> ()  [unwired: 8 in, 2 out]
        n188 = call <vilib>:"CTRE_Phoenix_MotorControl_SetSelectedSensorPosition.vi"("New Sensor Position"=0 ("New Position"), "PhoenixMotorControlDevRef"=w277) -> ()  [unwired: 8 in, 2 out]
      }
    }
    n189 = case shown="True" w228 {
      tunnel: w261 -> [_ w274]
      frame False {
      }
      frame True {
        n190 = call <vilib>:"CTRE_Phoenix_MotorControl_SetQuadraturePosition_Enhanced.vi"("New Position"="outer arm pivot zero (ticks)", "PhoenixMotorControlDevRef"=w274) -> ()  [unwired: 8 in, 2 out]
      }
    }
    n191 = Wait (ms)(milliseconds to wait=u32 30) -> ()  [unwired: 1 out]
    n192 = And(x=w221, y=w222) -> (x .and. y?=w220:bool)
    "safe_to_move_turret?" <- w220
    n193 = global write "Sensor_Values.vi" "Safe_To_Move_Turret?"(w220) -> ()
  }
  n194 = while {
    tunnel: w19 -> [w286]
    tunnel: w18 -> [w285]
    stop <- FALSE stop-if-true
    n195 = call <vilib>:"WPI_AnalogChannelGetVoltage.vi"("error in (no error)"=w285, "AIDeviceRef"=w286) -> ("Voltage"=w284:dbl)  [unwired: 7 in, 2 out]
    "Mag IR Voltage" <- w284
    n196 = Greater?(x=w284, y="mag IR threshold") -> (0:w282:bool)
    n197 = global write "Sensor_Values.vi" "Magazine_Loaded"(w282) -> ()
    n198 = Wait (ms)(milliseconds to wait=u32 30) -> ()  [unwired: 1 out]
  }
  n199 = while {
    stop <- FALSE stop-if-true
    n200 = global read "Calibration_And_Constant_Globals.vi" "Robot_Name"() -> (w290:enum16{"Alpha-2022", "Beta-2022"})
    n201 = case shown="\"Beta-2022\"" w290 {
      tunnel: ["limelight-alpha" ("Name") "limelight-beta" ("Name")] -> w289
      frame "Alpha-2022", Default {
      }
      frame "Beta-2022" {
      }
    }
    n202 = Concatenate Strings("/" ("string"), w289, "/" ("string")) -> (w301:string)
    n203 = Concatenate Strings(w301, "tx" ("Name")) -> (w304:string)
    n204 = Concatenate Strings(w301, "tv" ("Name")) -> (w292:string)
    n205 = Concatenate Strings(w301, "ty" ("Name")) -> (w300:string)
    n206 = call-poly <vilib>:"NT Read Value.vi"("Name"=w304) -> ("Numeric"=w310:dbl)  [unwired: 9 in, 1 out]
    n207 = call-poly <vilib>:"NT Read Value.vi"("Name"=w292) -> ("Boolean"=w291:bool)  [unwired: 9 in, 1 out]
    n208 = call-poly <vilib>:"NT Read Value.vi"("Name"=w300) -> ("Numeric"=w294:dbl)  [unwired: 9 in, 1 out]
    n209 = global write "Sensor_Values.vi" "Limelight_Has_Target?"(w291) -> ()
    n210 = global write "Sensor_Values.vi" "Camera_Goal_X (deg)"(w310) -> ()
    n211 = global write "Sensor_Values.vi" "Camera_Goal_Y (deg)"(w294) -> ()
    n212 = expression code="(x/180.0)*pi" "degrees to radians"(w294) -> (w293:dbl)
    n213 = expression code="(x/180.0)*pi" "degrees to radians"("limelight mounting angle (deg)") -> (w296:dbl)
    n214 = formula code="distance = (h2-h1) / tan(a1+a2);"("h2"="height of the target (in)", "h1"="height of robot (in)", "a1"=w296, "a2"=w293) -> ("distance"=w297:dbl)
    "limelight_distance_to_target" <- w297
    n215 = Wait (ms)(milliseconds to wait=u32 30) -> ()  [unwired: 1 out]
    n216 = global write "Sensor_Values.vi" "Limelight_Distance_To_Target (in)"(w297) -> ()
  }
  n217 = global read "Flywheel_Hardware_Globals.vi" "Flywheel_Left"() -> (w17:string)
  n218 = global read "Cowl_Hardware_Globals.vi" "Cowl Motor"() -> (w21:string)
  n219 = global read "Magazine_Globals.vi" "Magazine_Motor"() -> (w11:string)
  n220 = global read "Flywheel_Hardware_Globals.vi" "Flywheel_Right"() -> (w16:string)
  n221 = global read "Turret_Hardware_Globals.vi" "Turret_Ref"() -> (w6:string)
  n222 = call <vilib>:"CTRE_Phoenix_MotorControl_RefNumRegistryGet.vi"("refnum name"=w21) -> ("error out"=w8:errorcluster, "PhoenixMotorControlDevRef"=w7:T1)  [unwired: 9 in]
  n223 = call <vilib>:"CTRE_Phoenix_MotorControl_RefNumRegistryGet.vi"("refnum name"=w6) -> ("error out"=w4:errorcluster, "PhoenixMotorControlDevRef"=w5:T1)  [unwired: 9 in]
  n224 = call <vilib>:"CTRE_Phoenix_MotorControl_RefNumRegistryGet.vi"("refnum name"=w17) -> ("error out"=w14:errorcluster, "PhoenixMotorControlDevRef"=w15:T1)  [unwired: 9 in]
  n225 = call <vilib>:"CTRE_Phoenix_MotorControl_RefNumRegistryGet.vi"("refnum name"=w16) -> ("error out"=w12:errorcluster, "PhoenixMotorControlDevRef"=w13:T1)  [unwired: 9 in]
  n226 = call <vilib>:"CTRE_Phoenix_MotorControl_RefNumRegistryGet.vi"("refnum name"=w11) -> ("error out"=w9:errorcluster, "PhoenixMotorControlDevRef"=w10:T1)  [unwired: 9 in]
  n227 = while {
    tunnel: w7 -> [w316]
    tunnel: w8 -> [w327]
    stop <- FALSE stop-if-true
    w319 = 74.03 ("y")
    # "if 6479 is 45.6 degrees, and 2833 is 61.6 degrees, then find linear function using slope and initial condition\ny = -16/3646 x + 74.03"
    n228 = global read "Calibration_And_Constant_Globals.vi" "Zero_All"() -> (w314:bool)
    n229 = call-poly <vilib>:"CTRE_Phoenix_MotorController_Get_Enhanced.vi"("PhoenixMotorControlDevRef"=w316, "error in"=w327) -> ("Position (Raw Sensor Units)"=w326:i32)  [unwired: 10 in, 3 out]
    n230 = Compound Arithmetic op=OR("reset_cowl_position", w314) -> (w313:bool)
    n231 = case shown="True" w313 {
      tunnel: w316 -> [_ w331]
      frame False {
      }
      frame True {
        n232 = call <vilib>:"CTRE_Phoenix_MotorControl_SetQuadraturePosition_Enhanced.vi"("New Position"=0, "PhoenixMotorControlDevRef"=w331) -> ()  [unwired: 8 in, 2 out]
      }
    }
    n233 = Divide(x=-16.0, y=3646.0) -> (x/y=w324:dbl)
    n234 = Multiply(x=w326, y=w324) -> (x*y=w325:dbl)
    n235 = Add(x=w325, y=w319) -> (x+y=w321:dbl)
    n236 = Subtract(x="Cowl_Zero(deg)", y=w319) -> (x-y=w317:dbl)
    n237 = Wait (ms)(milliseconds to wait=u32 30) -> ()  [unwired: 1 out]
    n238 = Add(x=w321, y=w317) -> (x+y=w320:dbl)
    n239 = global write "Sensor_Values.vi" "Cowl_Angle(deg)"(w320) -> ()
  }
  n240 = while {
    tunnel: w15 -> [w348]
    tunnel: w14 -> [w347]
    tunnel: w13 -> [w346]
    tunnel: w12 -> [w345]
    stop <- FALSE stop-if-true
    # "convert from raw sensor units per 100 ms to RPM"
    n241 = call-poly <vilib>:"CTRE_Phoenix_MotorController_Get_TalonFX.vi"("PhoenixMotorControlDevRef"=w348, "error in"=w347) -> ("Velocity (Raw Sensor Units per 100 ms)"=w344:i32)  [unwired: 10 in, 3 out]
    n242 = call-poly <vilib>:"CTRE_Phoenix_MotorController_Get_TalonFX.vi"("PhoenixMotorControlDevRef"=w346, "error in"=w345) -> ("Velocity (Raw Sensor Units per 100 ms)"=w343:i32)  [unwired: 10 in, 3 out]
    n243 = Add(x=w344, y=w343) -> (x+y=w342:i32)
    n244 = Divide(x=w342, y=2) -> (x/y=w340:dbl)
    n245 = Divide(x=w340, y=2048) -> (x/y=w336:dbl)
    n246 = Multiply(x=w336, y=10.0) -> (x*y=w334:dbl)
    n247 = Multiply(x=w334, y=60.0) -> (x*y=w332:dbl)
    n248 = global write "Sensor_Values.vi" "Flywheel_Velocity(RPM)"(w332) -> ()
    n249 = Wait (ms)(milliseconds to wait=u32 30) -> ()  [unwired: 1 out]
  }
  n250 = while {
    tunnel: w10 -> [w351]
    tunnel: w9 -> [w350]
    stop <- FALSE stop-if-true
    n251 = call-poly <vilib>:"CTRE_Phoenix_MotorController_Get_Enhanced.vi"("PhoenixMotorControlDevRef"=w351, "error in"=w350) -> ("Velocity (Raw Sensor Units per 100 ms)"=w349:i32)  [unwired: 10 in, 3 out]
    n252 = global write "Sensor_Values.vi" "Magazine_Velocity(ticks/100ms)"(w349) -> ()
    n253 = Wait (ms)(milliseconds to wait=u32 30) -> ()  [unwired: 1 out]
  }
  n254 = while {
    tunnel: w5 -> [w357]
    tunnel: [w369] -> _
    tunnel: w4 -> [w369]
    stop <- FALSE stop-if-true
    # "dunno why the normal conversion doesn't work, this is our correction factor"
    n255 = global read "Calibration_And_Constant_Globals.vi" "Zero_All"() -> (w355:bool)
    n256 = call-poly <vilib>:"CTRE_Phoenix_MotorController_Get_Enhanced.vi"("PhoenixMotorControlDevRef"=w357, "error in"=w369) -> ("Position (Raw Sensor Units)"=w368:i32)  [unwired: 10 in, 3 out]
    "turret position" <- w368
    n257 = Compound Arithmetic op=OR("reset_turret_position", w355) -> (w354:bool)
    n258 = Divide(x=w368, y=4096) -> (x/y=w366:dbl)
    n259 = case shown="True" w354 {
      tunnel: w357 -> [_ w371]
      frame False {
      }
      frame True {
        n260 = call <vilib>:"CTRE_Phoenix_MotorControl_SetQuadraturePosition_Enhanced.vi"("New Position"=0, "PhoenixMotorControlDevRef"=w371) -> ()  [unwired: 8 in, 2 out]
      }
    }
    n261 = Divide(x=w366, y=572.43 ("x/y")) -> (x/y=w364:dbl)
    n262 = Multiply(x=w364, y=360.0) -> (x*y=w360:dbl)
    n263 = Multiply(x=w360, y=50.53) -> (x*y=w358:dbl)
    n264 = global write "Sensor_Values.vi" "Turret_Relative_Position(Degrees)"(w358) -> ()
    n265 = Wait (ms)(milliseconds to wait=u32 30) -> ()  [unwired: 1 out]
  }
